vi "Query S Parameters.vi"(8 "error in (no error)":errorcluster, 10 "Sparameters (string)":string[](array[string]), 11 "VNA-Keysight PNA in":refnum<class "VNA-Keysight PNA.lvclass">) -> (0 "error out":errorcluster, 2 "S parameters":T1[](array[typedef]), 3 "VNA-Keysight PNA out":refnum<class "VNA-Keysight PNA.lvclass">)   [LabVIEW 2020, in "VNA-Keysight PNA.lvclass"]
doc: "Queryes the S parameter choosen. It can give single parameter or full 2 to 4 port parameters.\nFor one port S Parameter array only have Sxx.\nFor N ports the S Parameter array hold S11,S12,...,S1N,S21,S22,...,SNN"
uses:
  VNA-Keysight PNA.lvclass
  C:/Sandbox/Git_Sandbox/WiSpry Test Framework source code (LV20)/WiSpry Test Framework/Instruments/Instrument.lvclass
  C:/Sandbox/Git_Sandbox/WiSpry Test Framework source code (LV20)/WiSpry Test Framework/Instruments/Vector Network Analyzer/Vector Network Analyzer.lvclass
  Controls/Sparameter cluster.ctl
  Vector Network Analyzer.lvclass/Vector Network Analyzer.ctl
  Instrument.lvclass/Instrument.ctl
  Instrument.lvclass
  Vector Network Analyzer.lvclass
panel:
  out "return count":u32
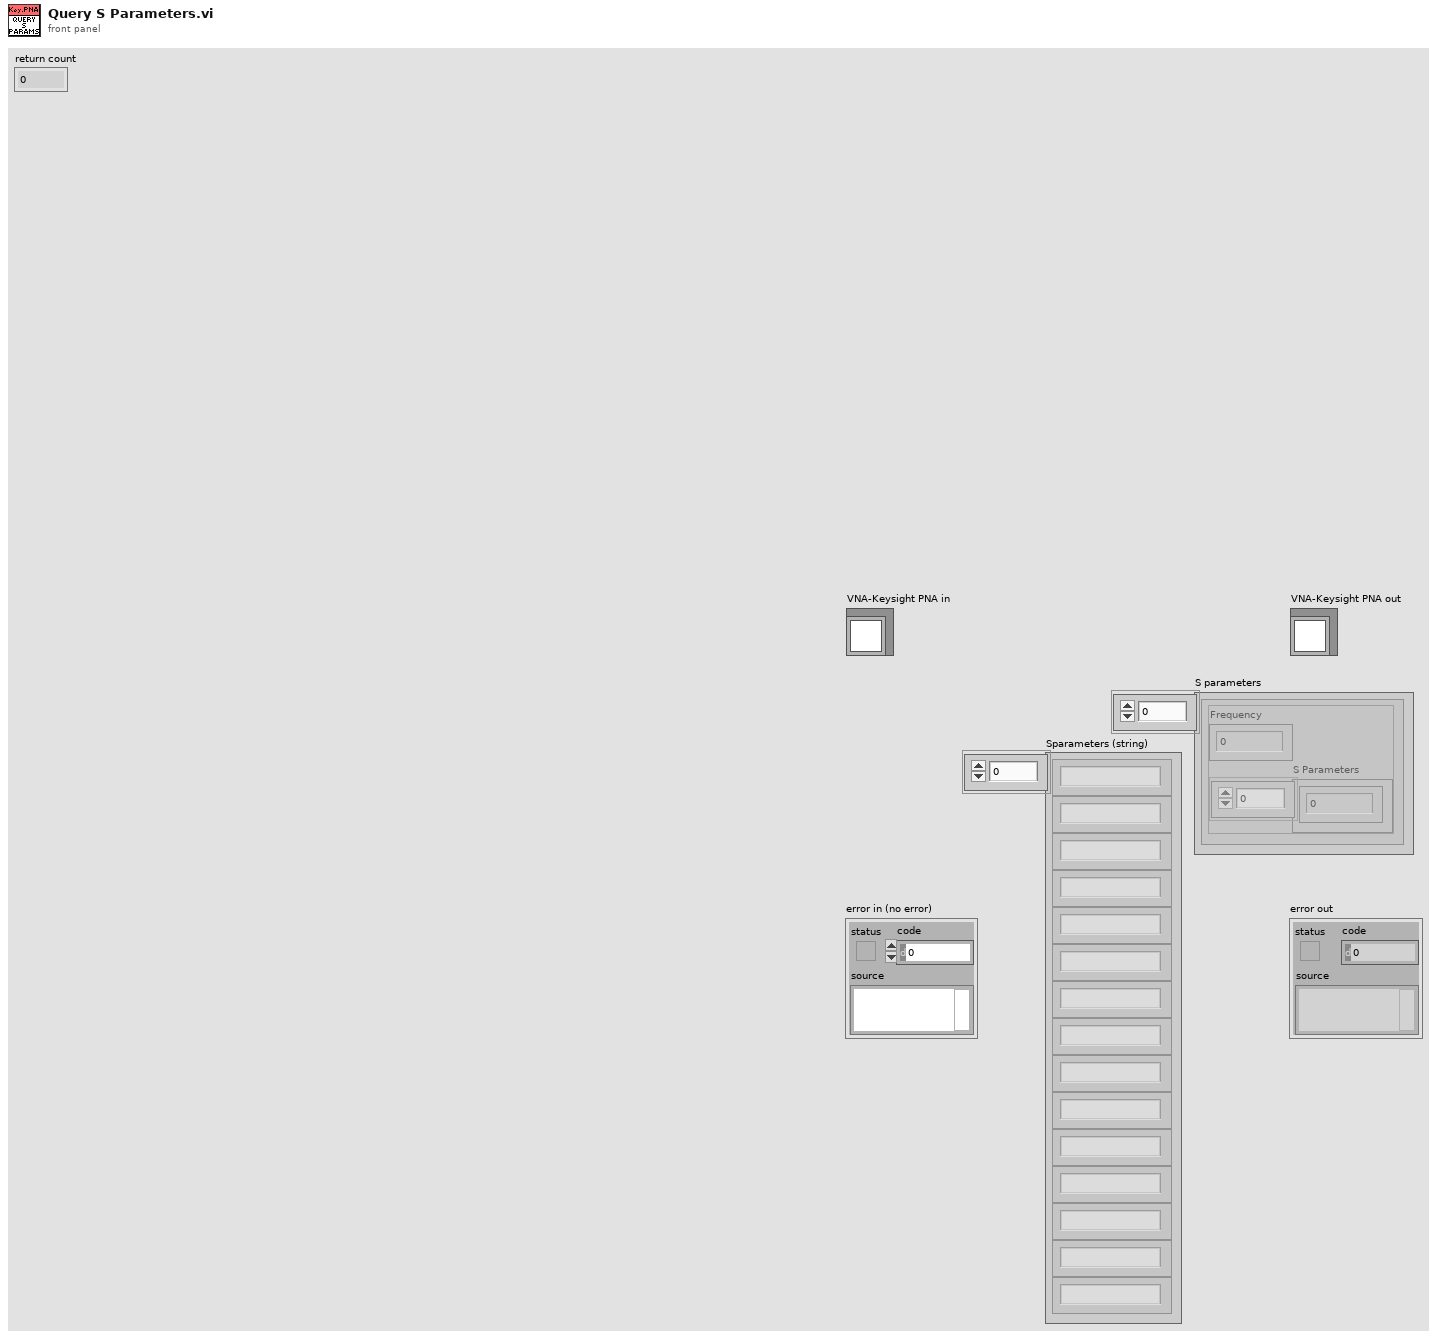
[diagram p1: front panel]
types:
  T1 = typedef "Vector Network Analyzer.lvclass/Sparameter cluster.ctl" = cluster{"Frequency":dbl, "S Parameters":cdb[]}
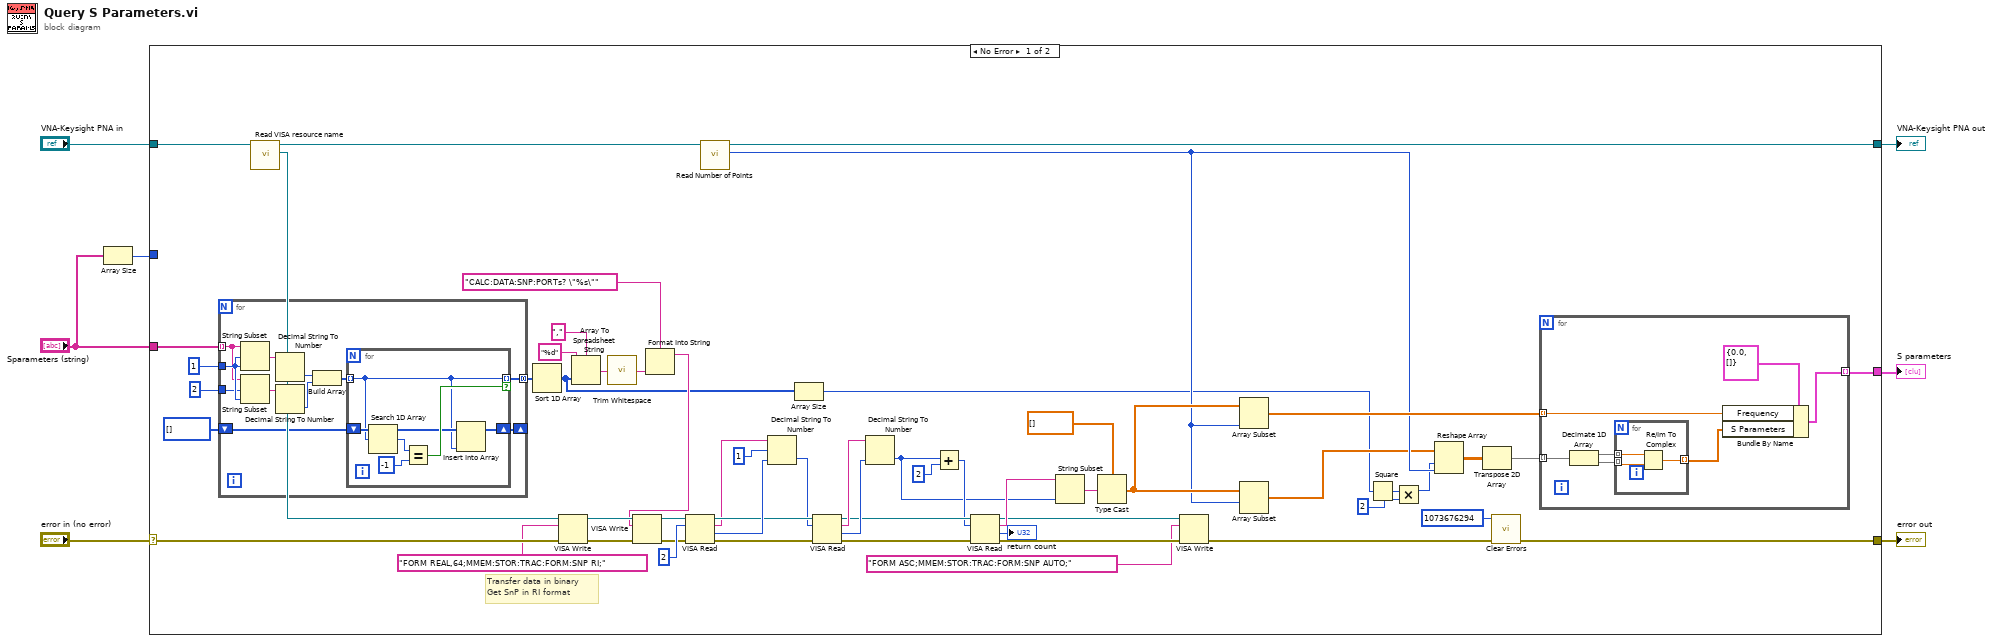
[diagram p0: block diagram]
diagram:
  n1 = Array Size(array="Sparameters (string)") -> (size(s)=w1:i32)
  n2 = case shown="No Error" "error in (no error)" {
    selector: "error in (no error)" -> [w63 w93]
    tunnel: w1 -> [_ _]
    tunnel: "VNA-Keysight PNA in" -> [w64 w92]
    tunnel: [w62 w92] -> w5
    tunnel: [w9 w93] -> w7
    tunnel: [w61 _] -> w6
    tunnel: "Sparameters (string)" -> [w22 _]
    frame No Error {
      # "Transfer data in binary\nGet SnP in RI format"
      n3 = for {
        tunnel: w22 -> [w71] mode=indexing
        tunnel: 1 ("offset (0)") -> [w75]
        tunnel: 2 ("offset (0)") -> [w74]
        tunnel: [w67] -> w18 mode=concatenating
        shift-right: [w65] -> _
        shift-left: i32[] [] -> [w68]
        n4 = String Subset(string=w71, offset (0)=w75, length (rest)=w75) -> (substring=w72:string)
        n5 = String Subset(string=w71, offset (0)=w74, length (rest)=w75) -> (substring=w73:string)
        n6 = Decimal String To Number(string=w72) -> (number=w69:i32)  [unwired: 2 in, 1 out]
        n7 = Decimal String To Number(string=w73) -> (number=w70:i32)  [unwired: 2 in, 1 out]
        n8 = Build Array(w69, w70) -> (w66:i32[])
        n9 = for {
          tunnel: w66 -> [w76] mode=indexing
          tunnel: [w76] -> w67 mode=indexing if=w79
          shift-right: [w77] -> w65
          shift-left: w68 -> [w78]
          n10 = Search 1D Array(1D array=w78, element=w76) -> (index of element=w81:i32)  [unwired: 1 in]
          n11 = Equal?(x=w81, y=-1) -> (x = y?=w79:bool)
          n12 = Insert Into Array(array=w78, new element=w76) -> (w77:i32[])  [unwired: 1 in]
        }
      }
      n13 = call "Read VISA resource name.vi"("Instrument in"=w64) -> ("VISA resource name"=w29:refnum<visa-resource-name>, "Instrument out"=w39:refnum<class "VNA-Keysight PNA.lvclass">)  [unwired: 9 in]
      n14 = Sort 1D Array(array=w18) -> (sorted array=w13:i32[])
      n15 = VISA Write(VISA resource name=w29, write buffer="FORM REAL,64;MMEM:STOR:TRAC:FORM:SNP RI;", error in (no error)=w63) -> (VISA resource name out=w58:refnum<visa-resource-name>, error out=w59:errorcluster)  [unwired: 1 out]
      n16 = Array To Spreadsheet String(delimiter (Tab)=",", array=w13, 3:"%d" ("format string")) -> (spreadsheet string=w15:string)
      n17 = call <vilib>:"Trim Whitespace.vi"("string"=w15) -> ("trimmed string"=w14:string)  [unwired: 1 in]
      n18 = Format Into String(format string="CALC:DATA:SNP:PORTs? \"%s\"", w14) -> (resulting string=w57:string)  [unwired: 2 in, 1 out]
      n19 = VISA Write(VISA resource name=w58, write buffer=w57, error in (no error)=w59) -> (VISA resource name out=w45:refnum<visa-resource-name>, error out=w46:errorcluster)  [unwired: 1 out]
      n20 = VISA Read(VISA resource name=w45, byte count=u32 2, error in (no error)=w46) -> (VISA resource name out=w54:refnum<visa-resource-name>, read buffer=w36:string, return count=w55:u32, error out=w10:errorcluster)
      n21 = call "Read Number of Points.vi"("Vector Network Analyzer in"=w39) -> ("Number of Points"=w31:i32, "Vector Network Analyzer out"=w62:refnum<class "VNA-Keysight PNA.lvclass">)  [unwired: 9 in]
      n22 = Decimal String To Number(string=w36, offset=1 ("offset (0)"), default (0L)=w55) -> (number=w53:u32)  [unwired: 1 out]
      n23 = Array Size(array=w13) -> (size(s)=w12:i32)
      n24 = VISA Read(VISA resource name=w54, byte count=w53, error in (no error)=w10) -> (VISA resource name out=w49:refnum<visa-resource-name>, read buffer=w51:string, return count=w50:u32, error out=w47:errorcluster)
      n25 = Decimal String To Number(string=w51, default (0L)=w50) -> (number=w40:u32)  [unwired: 1 in, 1 out]
      n26 = Add(x=w40, y=u32 2) -> (x+y=w48:u32)
      n27 = VISA Read(VISA resource name=w49, byte count=w48, error in (no error)=w47) -> (VISA resource name out=w42:refnum<visa-resource-name>, read buffer=w44:string, return count=→"return count":u32, error out=w43:errorcluster)
      n28 = String Subset(string=w44, length (rest)=w40) -> (substring=w34:string)  [unwired: 1 in]
      n29 = Type Cast(type=dbl[] [], x=w34) -> (*(type *) &x=w33:dbl[])
      n30 = VISA Write(VISA resource name=w42, write buffer="FORM ASC;MMEM:STOR:TRAC:FORM:SNP AUTO;", error in (no error)=w43) -> (error out=w8:errorcluster)  [unwired: 2 out]
      n31 = Array Subset(array=w33, length=w31) -> (w38:dbl[])  [unwired: 1 in]
      n32 = Array Subset(array=w33, index=w31) -> (w27:dbl[])  [unwired: 1 in]
      n33 = Square(x=w12) -> (x^2=w32:i32)
      n34 = Multiply(x=w32, y=2) -> (x*y=w26:i32)
      n35 = Reshape Array(w27, w26, w31) -> (w28:dbl[][])
      n36 = Transpose 2D Array(2D array=w28) -> (transposed array=w30:dbl[][])
      n37 = call <vilib>:"Clear Errors.vi"("error in (no error)"=w8, "specific error code to clear (0: all)"=1073676294) -> ("error out"=w9:errorcluster)  [unwired: 4 in, 1 out]
      n38 = for {
        tunnel: w38 -> [w86] mode=indexing
        tunnel: w30 -> [w85] mode=indexing
        tunnel: [w87] -> w61 mode=indexing
        n39 = Decimate 1D Array(w85) -> (w84:dbl[], w83:dbl[])
        n40 = for {
          tunnel: w84 -> [w91] mode=indexing
          tunnel: w83 -> [w90] mode=indexing
          tunnel: [w89] -> w82 mode=indexing
          n41 = Re/Im To Complex(1:w90, 2:w91) -> (0:w89:cdb)
        }
        n42 = Bundle By Name(cluster=T1 {"Frequency"=0.0, "S Parameters"=[]} ("S Parameters"), "Frequency"=w86, "S Parameters"=w82) -> (w87:T1)
      }
    }
    frame Error {
    }
  }
  "error out" <- w7
  "VNA-Keysight PNA out" <- w5
  "S parameters" <- w6
